vi "Construct.vi"   [LabVIEW 2019, in "SQLite Database.lvclass"]
doc: "Polymorphic, selectable constructor for a SQLite Database sink.\n\n<b>Code Developed By:</b>\nTechnology Service Corporation\nBloomington, IN 47403\nwww.tsc.com/atcs\n\nDeveloper:\nDaniel Coons"
uses:
  SQLite Database.lvclass
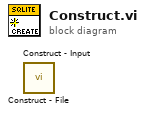
[diagram p0: block diagram]
diagram:
  n1 = call "Construct - Input.vi"() -> ()  [unwired: 10 in, 2 out]
  n2 = call "Construct - File.vi"() -> ()  [unwired: 10 in, 2 out]
